vi "Write CAN Frame in CVT.vi"(8 "error in (no error)":errorcluster, 11 "CAN Frame":string[][](array[string])) -> (0 "error out":errorcluster)   [LabVIEW 2021, in "CAN.lvlib"]
uses:
  CAN.lvlib
  Support Libraries/Current Value Table/Type Defs/Group Data.ctl
  Support Libraries/Current Value Table/Write grouped data to tags.vi
  Support Libraries/Current Value Table/Write Index Set.vi
  Support Libraries/Current Value Table/DataTypes/Double_Write Index Set.vi
  Support Libraries/Current Value Table/DataTypes/Array of String_Write Index Set.vi
  Support Libraries/Current Value Table/DataTypes/Array of Boolean_Write Index Set.vi
  Support Libraries/Current Value Table/DataTypes/Array of Single_Write Index Set.vi
  Support Libraries/Current Value Table/DataTypes/Array of Double_Write Index Set.vi
  Support Libraries/Current Value Table/DataTypes/Array of I8_Write Index Set.vi
  Support Libraries/Current Value Table/DataTypes/Array of I16_Write Index Set.vi
  Support Libraries/Current Value Table/DataTypes/Array of I32_Write Index Set.vi
  Support Libraries/Current Value Table/DataTypes/Array of I64_Write Index Set.vi
  Support Libraries/Current Value Table/DataTypes/Array of U64_Write Index Set.vi
  Support Libraries/Current Value Table/DataTypes/Array of U32_Write Index Set.vi
  Support Libraries/Current Value Table/DataTypes/Array of U16_Write Index Set.vi
  Support Libraries/Current Value Table/DataTypes/Array of U8_Write Index Set.vi
  Support Libraries/Current Value Table/DataTypes/Boolean_Write Index Set.vi
  Support Libraries/Current Value Table/DataTypes/String_Write Index Set.vi
  Support Libraries/Current Value Table/DataTypes/U8_Write Index Set.vi
  Support Libraries/Current Value Table/DataTypes/U16_Write Index Set.vi
  Support Libraries/Current Value Table/DataTypes/U32_Write Index Set.vi
  Support Libraries/Current Value Table/DataTypes/U64_Write Index Set.vi
  Support Libraries/Current Value Table/DataTypes/I8_Write Index Set.vi
  Support Libraries/Current Value Table/DataTypes/I16_Write Index Set.vi
  Support Libraries/Current Value Table/DataTypes/I32_Write Index Set.vi
  Support Libraries/Current Value Table/DataTypes/I64_Write Index Set.vi
  Support Libraries/Current Value Table/DataTypes/Single_Write Index Set.vi
  Support Libraries/Current Value Table/FGVs/Group Memory.vi
  Support Libraries/Current Value Table/Memory Block.vi
  Support Libraries/Current Value Table/DataTypes/Double_Memory Block.vi
  Support Libraries/Current Value Table/DataTypes/Array of String_Memory Block.vi
  Support Libraries/Current Value Table/DataTypes/Array of Boolean_Memory Block.vi
  Support Libraries/Current Value Table/DataTypes/Array of Single_Memory Block.vi
  Support Libraries/Current Value Table/DataTypes/Array of Double_Memory Block.vi
  Support Libraries/Current Value Table/DataTypes/Array of I8_Memory Block.vi
  Support Libraries/Current Value Table/DataTypes/Array of I16_Memory Block.vi
  Support Libraries/Current Value Table/DataTypes/Array of I32_Memory Block.vi
  Support Libraries/Current Value Table/DataTypes/Array of I64_Memory Block.vi
  Support Libraries/Current Value Table/DataTypes/Array of U64_Memory Block.vi
  Support Libraries/Current Value Table/DataTypes/Array of U32_Memory Block.vi
  Support Libraries/Current Value Table/DataTypes/Array of U16_Memory Block.vi
  Support Libraries/Current Value Table/DataTypes/Array of U8_Memory Block.vi
  Support Libraries/Current Value Table/DataTypes/Boolean_Memory Block.vi
  Support Libraries/Current Value Table/DataTypes/String_Memory Block.vi
  Support Libraries/Current Value Table/DataTypes/U8_Memory Block.vi
  Support Libraries/Current Value Table/DataTypes/U16_Memory Block.vi
  Support Libraries/Current Value Table/DataTypes/U32_Memory Block.vi
  Support Libraries/Current Value Table/DataTypes/U64_Memory Block.vi
  Support Libraries/Current Value Table/DataTypes/I8_Memory Block.vi
  Support Libraries/Current Value Table/DataTypes/I16_Memory Block.vi
  Support Libraries/Current Value Table/DataTypes/I32_Memory Block.vi
  Support Libraries/Current Value Table/DataTypes/I64_Memory Block.vi
  Support Libraries/Current Value Table/DataTypes/Single_Memory Block.vi
  Support Libraries/Current Value Table/Current Value Table.lvlib
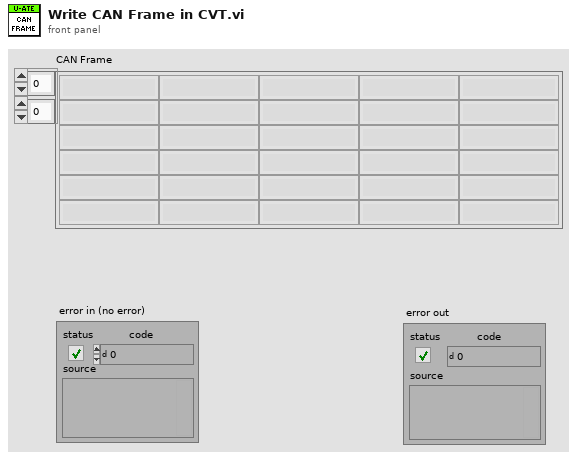
[diagram p1: front panel]
types:
  T1 = typedef "CVT.lvlib/Current Value Table.lvlib/Group Data.ctl" = cluster{"Double":dbl[], "Single":sgl[], "I64":i64[], "I32":i32[], "I16":i16[], "I8":i8[], "U64":u64[], "U32":u32[], "U16":u16[], "U8":u8[], "String":string[], "Boolean":bool[], "Array of U8":cluster{"U8 Array":u8[]}[], "Array of U16":cluster{"U16 Array":u16[]}[], "Array of U32":cluster{"U32 Array":u32[]}[], "Array of U64":cluster{"U64 Array":u64[]}[], "Array of I64":cluster{"I64 Array":i64[]}[], "Array of I32":cluster{"I32 Array":i32[]}[], "Array of I16":cluster{"I16 Array":i16[]}[], "Array of I8":cluster{"I8 Array":i8[]}[], "Array of Double":cluster{"DBL Array":dbl[]}[], "Array of Single":cluster{"SGL Array":sgl[]}[], "Array of Boolean":cluster{"Boolean Array":bool[]}[], "Array of String":cluster{"String Array":string[]}[]}
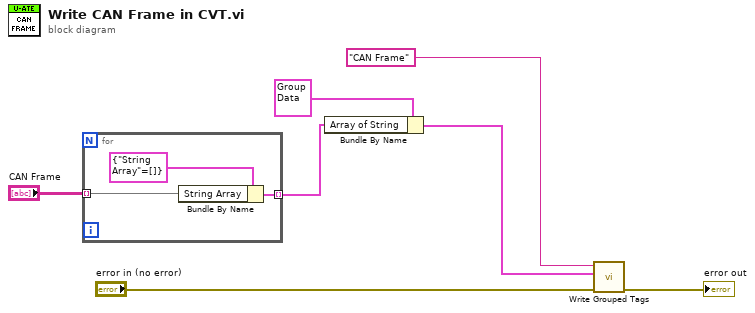
[diagram p0: block diagram]
diagram:
  n1 = for {
    tunnel: "CAN Frame" -> [w9] mode=indexing
    tunnel: [w8] -> w3 mode=indexing
    n2 = Bundle By Name(cluster=cluster{"String Array":string[]} {"String Array"=[]} ("DummyStringArrayCluster"), "String Array"=w9) -> (w8:cluster{"String Array":string[]})
  }
  n3 = Bundle By Name(cluster=T1 {"Double"=[], "Single"=[], "I64"=[], "I32"=[], "I16"=[], "I8"=[], "U64"=[], "U32"=[], "U16"=[], "U8"=[], "String"=[], "Boolean"=[], "Array of U8"=[], "Array of U16"=[], "Array of U32"=[], "Array of U64"=[], "Array of I64"=[], "Array of I32"=[], "Array of I16"=[], "Array of I8"=[], "Array of Double"=[], "Array of Single"=[], "Array of Boolean"=[], "Array of String"=[]} ("Data"), "Array of String"=w3) -> (w4:T1)
  n4 = call "Write Grouped Tags.vi"("error in (no error)"="error in (no error)", "Data"=w4, "Group"="CAN Frame") -> ("error out"=→"error out":errorcluster)  [unwired: 8 in]
